vi "Graph Utilities Tree 2.vi"() -> ()   [LabVIEW 2016]
uses:
  graph_utilities.lvclass
panel:
  out "XY Graph":cluster{"Intensity Data":dbl[], "Array":dbl[]}[](graph)
  out "Intensity Graph":dbl[][](graph)
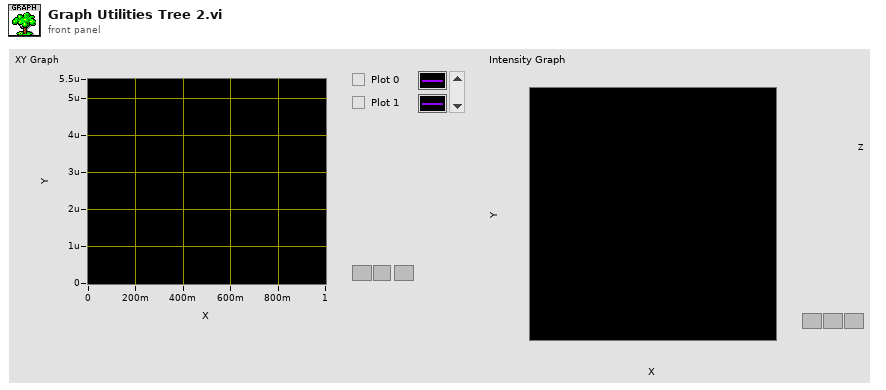
[diagram p1: front panel]
types:
  T1 = typedef "LVPointDoubleTypeDef.ctl" = cluster{"X":dbl, "Y":dbl}
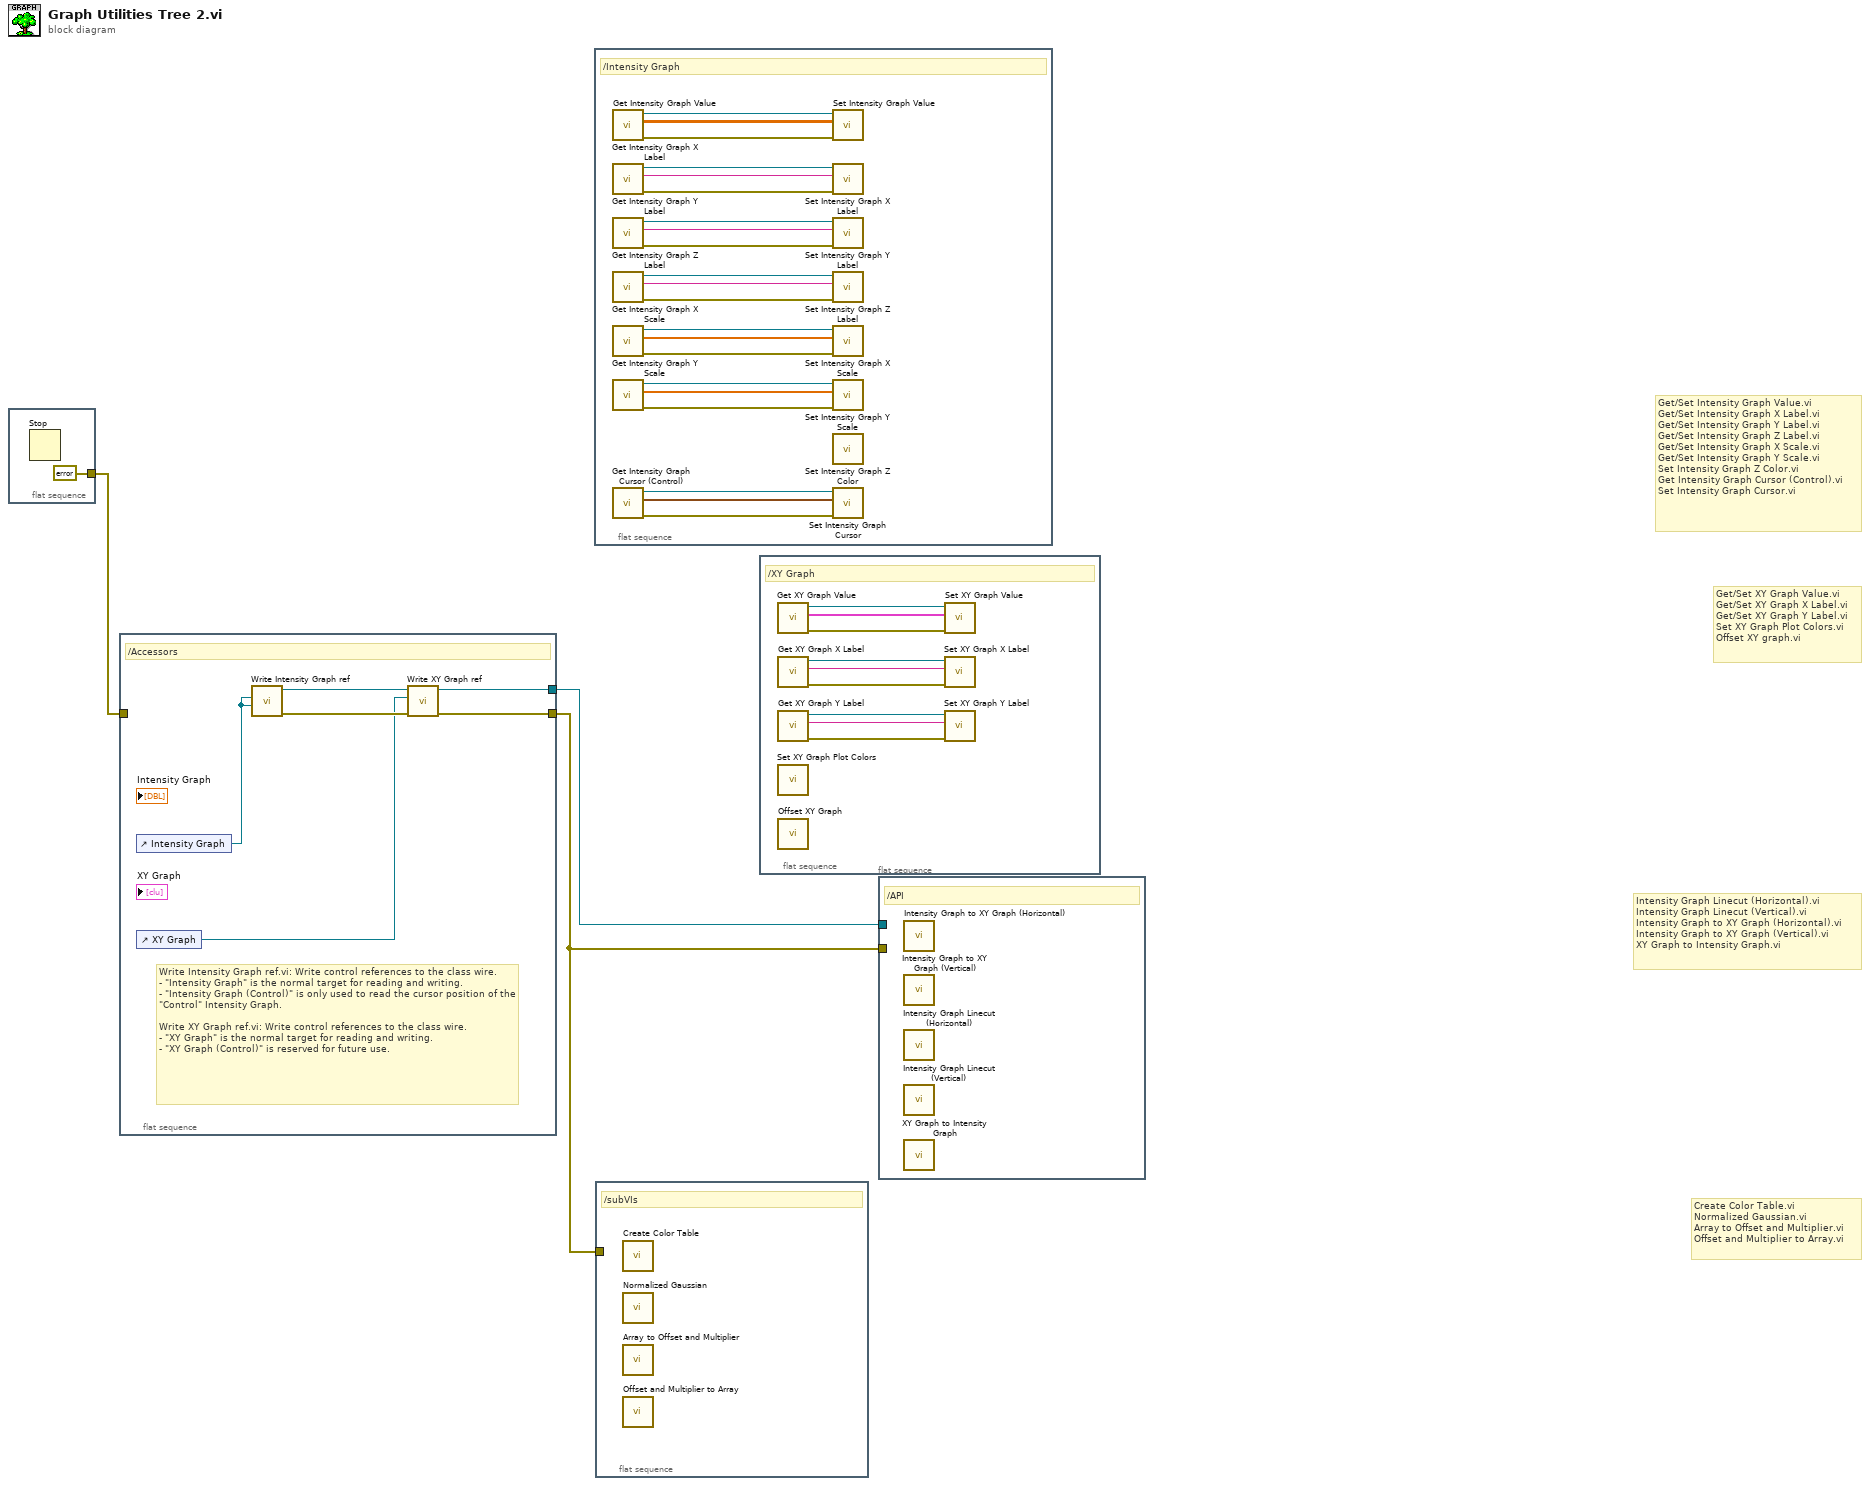
[diagram p0: block diagram]
diagram:
  # "Create Color Table.vi\nNormalized Gaussian.vi\nArray to Offset and Multiplier.vi\nOffset and Multiplier to Array.vi"
  # "Get/Set Intensity Graph Value.vi\nGet/Set Intensity Graph X Label.vi\nGet/Set Intensity Graph Y Label.vi\nGet/Set Intensity Graph Z Label.vi\nGet/Set Intensity Graph X Scale.vi\nGet/Set Intensity Graph Y Scale.vi\nSet Intensity Graph Z Color.vi\nGet Intensity Graph Cursor (Control).vi\nSet Intensity Graph Cursor.vi"
  # "Get/Set XY Graph Value.vi\nGet/Set XY Graph X Label.vi\nGet/Set XY Graph Y Label.vi\nSet XY Graph Plot Colors.vi\nOffset XY graph.vi"
  # "Intensity Graph Linecut (Horizontal).vi\nIntensity Graph Linecut (Vertical).vi\nIntensity Graph to XY Graph (Horizontal).vi\nIntensity Graph to XY Graph (Vertical).vi\nXY Graph to Intensity Graph.vi"
  n1 = flat-sequence {
    tunnel: [errorcluster {"status"=FALSE, "code"=0, "source"=""} ("error in (no error)")] -> w3
    frame #0 {
      n2 = Stop() -> ()  [unwired: 1 in]
    }
  }
  n3 = flat-sequence {
    tunnel: w3 -> [_]
    tunnel: [w7] -> w2
    tunnel: [w6] -> w1
    frame #0 {
      # "Write Intensity Graph ref.vi: Write control references to the class wire.\n- \"Intensity Graph\" is the normal target for reading and writing.\n- \"Intensity Graph (Control)\" is only used to read the cursor position of the \"Control\" Intensity Graph.\n\nWrite XY Graph ref.vi: Write control references to the class wire.\n- \"XY Graph\" is the normal target for reading and writing.\n- \"XY Graph (Control)\" is reserved for future use."
      # "/Accessors"
      n4 = control-ref of="Intensity Graph"() -> (w8:refnum<vi>)
      n5 = control-ref of="XY Graph"() -> (w5:refnum<vi>)
      n6 = call "Write Intensity Graph ref.vi"("Intensity Graph (Control)"=w8, "Intensity Graph"=w8) -> ("error out"=w9:errorcluster, "graph_utilities out"=w10:refnum<class "graph_utilities.lvclass">)  [unwired: 8 in]
      n7 = call "Write XY Graph ref.vi"("error in (no error)"=w9, "XY Graph"=w5, "graph_utilities in"=w10) -> ("error out"=w6:errorcluster, "graph_utilities out"=w7:refnum<class "graph_utilities.lvclass">)  [unwired: 7 in]
    }
  }
  n8 = flat-sequence {
    frame #0 {
      # "/Intensity Graph"
      n9 = call "Get Intensity Graph Value.vi"() -> ("error out"=w29:errorcluster, "Value"=w31:dbl[][], "graph_utilities out"=w30:refnum<class "graph_utilities.lvclass">)  [unwired: 9 in]
      n10 = call "Get Intensity Graph X Label.vi"() -> ("error out"=w27:errorcluster, "X Label"=w18:string, "graph_utilities out"=w28:refnum<class "graph_utilities.lvclass">)  [unwired: 9 in]
      n11 = call "Get Intensity Graph Y Label.vi"() -> ("error out"=w25:errorcluster, "Y Label"=w17:string, "graph_utilities out"=w26:refnum<class "graph_utilities.lvclass">)  [unwired: 9 in]
      n12 = call "Get Intensity Graph Z Label.vi"() -> ("error out"=w23:errorcluster, "Z Label"=w16:string, "graph_utilities out"=w24:refnum<class "graph_utilities.lvclass">)  [unwired: 9 in]
      n13 = call "Get Intensity Graph X Scale.vi"() -> ("error out"=w21:errorcluster, "X Scale"=w15:dbl[], "graph_utilities out"=w22:refnum<class "graph_utilities.lvclass">)  [unwired: 8 in, 1 out]
      n14 = call "Get Intensity Graph Y Scale.vi"() -> ("error out"=w19:errorcluster, "Y Scale"=w14:dbl[], "graph_utilities out"=w20:refnum<class "graph_utilities.lvclass">)  [unwired: 8 in, 1 out]
      n15 = call "Get Intensity Graph Cursor (Control).vi"() -> ("error out"=w12:errorcluster, "Cursor.Cursor Position"=w13:T1, "graph_utilities out"=w11:refnum<class "graph_utilities.lvclass">)  [unwired: 9 in]
      n16 = call "Set Intensity Graph Value.vi"("error in (no error)"=w29, "Value"=w31, "graph_utilities in"=w30) -> ()  [unwired: 7 in, 2 out]
      n17 = call "Set Intensity Graph X Label.vi"("error in (no error)"=w27, "X Label"=w18, "graph_utilities in"=w28) -> ()  [unwired: 7 in, 2 out]
      n18 = call "Set Intensity Graph Y Label.vi"("error in (no error)"=w25, "Y Label"=w17, "graph_utilities in"=w26) -> ()  [unwired: 7 in, 2 out]
      n19 = call "Set Intensity Graph Z Label.vi"("error in (no error)"=w23, "Z Label"=w16, "graph_utilities in"=w24) -> ()  [unwired: 7 in, 2 out]
      n20 = call "Set Intensity Graph X Scale.vi"("error in (no error)"=w21, "X Scale"=w15, "graph_utilities in"=w22) -> ()  [unwired: 7 in, 2 out]
      n21 = call "Set Intensity Graph Y Scale.vi"("error in (no error)"=w19, "Y Scale"=w14, "graph_utilities in"=w20) -> ()  [unwired: 7 in, 2 out]
      n22 = call "Set Intensity Graph Z Color.vi"() -> ()  [unwired: 10 in, 2 out]
      n23 = call "Set Intensity Graph Cursor.vi"("error in (no error)"=w12, "Cursor.Cursor Position"=w13, "graph_utilities in"=w11) -> ()  [unwired: 7 in, 2 out]
    }
  }
  n24 = flat-sequence {
    tunnel: w1 -> [_]
    frame #0 {
      # "/subVIs"
      n25 = call "Create Color Table.vi"() -> ()  [unwired: 2 in, 4 out]
      n26 = call "Normalized Gaussian.vi"() -> ()  [unwired: 10 in, 2 out]
      n27 = call "Array to Offset and Multiplier.vi"() -> ()  [unwired: 1 in, 1 out]
      n28 = call "Offset and Multiplier to Array.vi"() -> ()  [unwired: 2 in, 1 out]
    }
  }
  n29 = flat-sequence {
    frame #0 {
      # "/XY Graph"
      n30 = call "Get XY Graph Value.vi"() -> ("error out"=w38:errorcluster, "Value"=w40:cluster{dbl[], dbl[]}[], "graph_utilities out"=w39:refnum<class "graph_utilities.lvclass">)  [unwired: 9 in]
      n31 = call "Get XY Graph X Label.vi"() -> ("error out"=w36:errorcluster, "X Label"=w32:string, "graph_utilities out"=w37:refnum<class "graph_utilities.lvclass">)  [unwired: 9 in]
      n32 = call "Get XY Graph Y Label.vi"() -> ("error out"=w34:errorcluster, "Y Label"=w33:string, "graph_utilities out"=w35:refnum<class "graph_utilities.lvclass">)  [unwired: 9 in]
      n33 = call "Set XY Graph Plot Colors.vi"() -> ()  [unwired: 10 in, 2 out]
      n34 = call "Offset XY Graph.vi"() -> ()  [unwired: 10 in, 2 out]
      n35 = call "Set XY Graph Value.vi"("error in (no error)"=w38, "Value"=w40, "graph_utilities in"=w39) -> ()  [unwired: 7 in, 2 out]
      n36 = call "Set XY Graph X Label.vi"("error in (no error)"=w36, "X Label"=w32, "graph_utilities in"=w37) -> ()  [unwired: 7 in, 2 out]
      n37 = call "Set XY Graph Y Label.vi"("error in (no error)"=w34, "Y Label"=w33, "graph_utilities in"=w35) -> ()  [unwired: 7 in, 2 out]
    }
  }
  n38 = flat-sequence {
    tunnel: w2 -> [_]
    tunnel: w1 -> [_]
    frame #0 {
      # "/API"
      n39 = call "Intensity Graph to XY Graph (Horizontal).vi"() -> ()  [unwired: 10 in, 2 out]
      n40 = call "Intensity Graph to XY Graph (Vertical).vi"() -> ()  [unwired: 10 in, 2 out]
      n41 = call "Intensity Graph Linecut (Horizontal).vi"() -> ()  [unwired: 10 in, 2 out]
      n42 = call "Intensity Graph Linecut (Vertical).vi"() -> ()  [unwired: 10 in, 2 out]
      n43 = call "XY Graph to Intensity Graph.vi"() -> ()  [unwired: 10 in, 2 out]
    }
  }
